vi "extract_XML_string_between_start_end-2.vi"(10 "type":string, 11 "XML_Cluster_String in":string) -> (0 "InTagDefines":T1(array[cluster]), 1 "XML_between_startANDEnd":string, 2 "nesting_level":i32, 3 "XML_after_start_end_pair":string)   [LabVIEW 2011]
doc: "This VI will return the content between a start and end demarkation in XML finding the appropriate pair even when nested within another of the same type. As and example\n\nhello not this\n<device>\n this\n <device>\n more more more\n </device>\n and this\n</device>\nnot this \n\nwill return:\n this\n <device>\n more more more\n </device>\n and this\n\n\nit will omit the start and end strings."
uses:
  <vilib>/regexp/Match Regular Expression.xnode
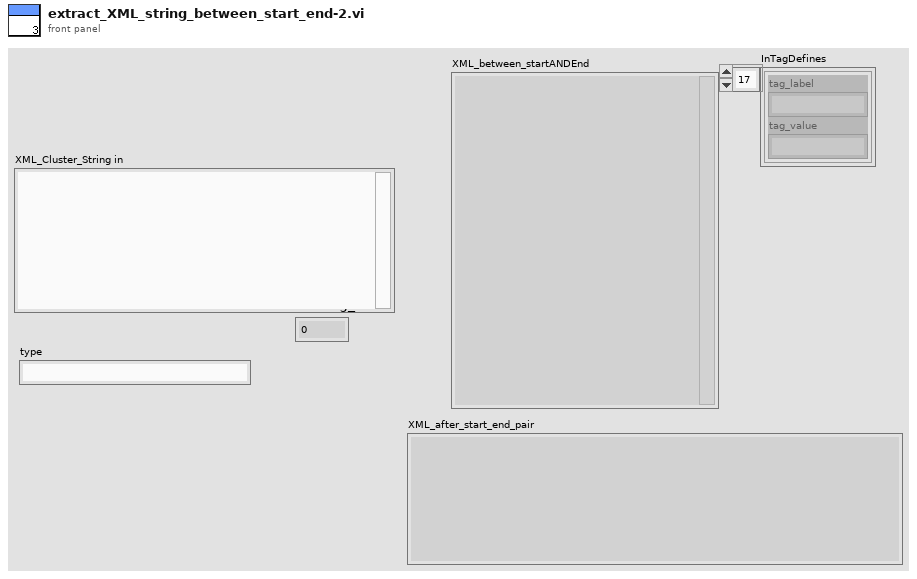
[diagram p1: front panel]
types:
  T1 = cluster{"tag_label":string, "tag_value":string}[]
  T2 = cluster{"submatch 1":string, "submatch 2":string}[]
  T3 = cluster{"submatch 1":string, "submatch 2":string}
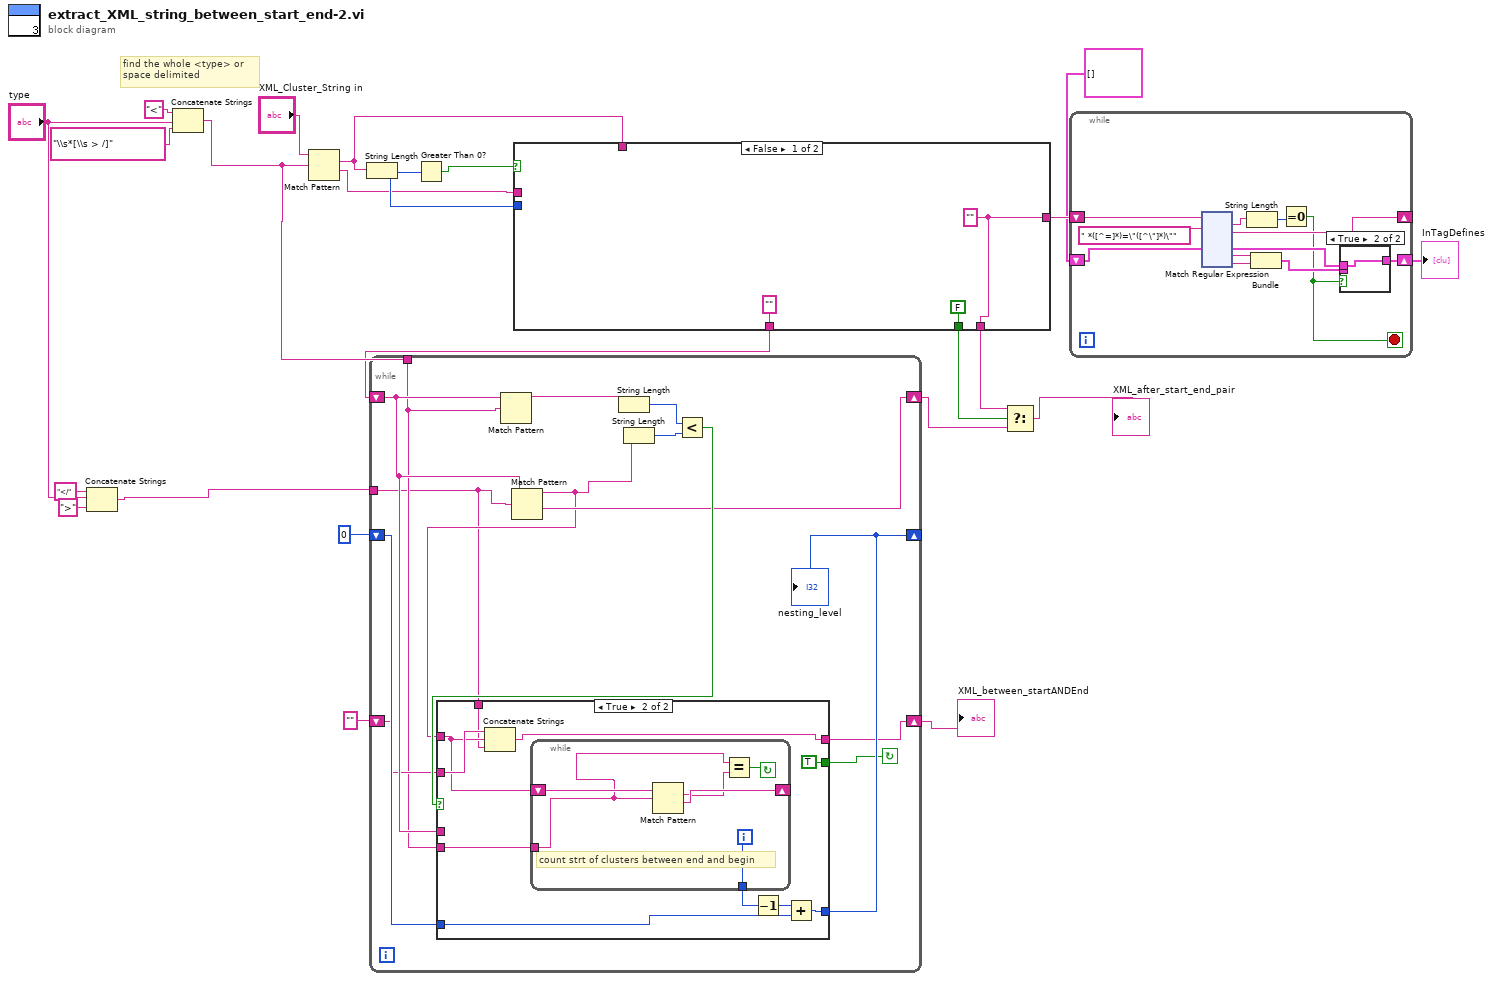
[diagram p0: block diagram]
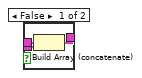
[diagram p2: hidden frame]
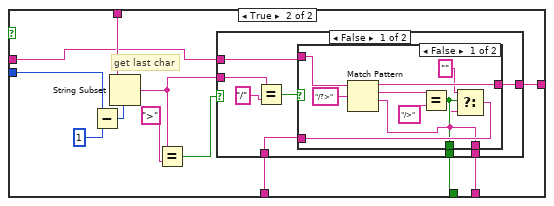
[diagram p3: hidden frame]
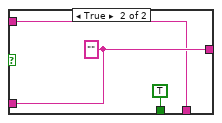
[diagram p4: hidden frame]
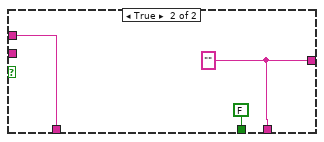
[diagram p5: hidden frame]
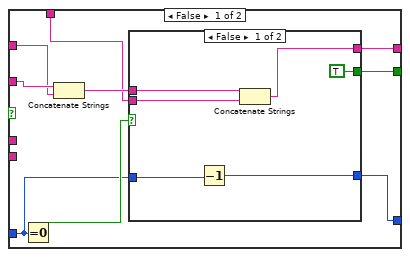
[diagram p6: hidden frame]
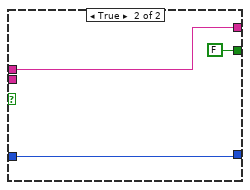
[diagram p7: hidden frame]
diagram:
  # "find the whole <type> or \nspace delimited"
  n1 = Concatenate Strings("</" ("string"), "type", ">" ("string")) -> (w21:string)
  n2 = Concatenate Strings("<" ("string"), "type", "\\s*[\\s > /]" ("string")) -> (w20:string)
  n3 = Match Pattern(string="XML_Cluster_String in", regular expression=w20) -> (match substring=w14:string, after substring=w9:string)  [unwired: 1 in, 2 out]
  n4 = String Length(string=w14) -> (length=w13:i32)
  n5 = Greater Than 0?(x=w13) -> (x > 0?=w10:bool)
  n6 = case shown="False" w10 {
    tunnel: w14 -> [_ w38]
    tunnel: w13 -> [_ w37]
    tunnel: w9 -> [_ w32]
    tunnel: ["" ("XML_Cluster_String in") w31] -> w8
    tunnel: [w24 w29] -> w7
    tunnel: [FALSE w28] -> w2
    tunnel: [w24 w27] -> w1
    frame False {
      w24 = "" ("XML_Cluster_String in")
    }
    frame True {
      # "get last char"
      n7 = Subtract(x=w37, y=1) -> (x-y=w35:i32)
      n8 = String Subset(string=w38, offset (0)=w35) -> (substring=w30:string)  [unwired: 1 in]
      n9 = Equal?(x=w30, y=">") -> (x = y?=w33:bool)
      n10 = case shown="False" w33 {
        tunnel: w32 -> [w44 w61]
        tunnel: [w43 w61] -> w31
        tunnel: w30 -> [w46 _]
        tunnel: [w42 w59] -> w29
        tunnel: [w40 FALSE] -> w28
        tunnel: [w39 w59] -> w27
        frame False {
          n11 = Equal?(x=w46, y="/") -> (x = y?=w41:bool)
          n12 = case shown="False" w41 {
            tunnel: w44 -> [w55 w56]
            tunnel: [w50 w58] -> w43
            tunnel: [w53 w58] -> w42
            tunnel: [w49 TRUE] -> w40
            tunnel: [w47 w56] -> w39
            frame False {
              n13 = Match Pattern(string=w55, regular expression="/?>") -> (before substring=w53:string, match substring=w52:string, after substring=w47:string)  [unwired: 1 in, 1 out]
              n14 = Equal?(x=w52, y="/>") -> (x = y?=w49:bool)
              n15 = Select(t="", s=w49, f=w47) -> (s? t:f=w50:string)
            }
            frame True {
              w58 = "" ("XML_Cluster_String in")
            }
          }
        }
        frame True {
          w59 = "" ("XML_Cluster_String in")
        }
      }
    }
  }
  n16 = while {
    shift-right: [w68] -> w3
    shift-left: w8 -> [w67]
    shift-right: [w70] -> _
    shift-left: 0 -> [w71]
    shift-right: [w64] -> w22
    shift-left: "" ("after substring") -> [w65]
    tunnel: w20 -> [w63]
    tunnel: w21 -> [w62]
    stop <- w69 continue-if-true
    n17 = Match Pattern(string=w67, regular expression=w63) -> (before substring=w75:string)  [unwired: 1 in, 3 out]
    n18 = Match Pattern(string=w67, regular expression=w62) -> (before substring=w66:string, after substring=w68:string)  [unwired: 1 in, 2 out]
    n19 = String Length(string=w75) -> (length=w74:i32)
    n20 = String Length(string=w66) -> (length=w73:i32)
    n21 = Less?(x=w74, y=w73) -> (x < y?=w72:bool)
    n22 = case shown="True" w72 {
      tunnel: w66 -> [w81 w99]
      tunnel: w71 -> [w78 w103]
      tunnel: [w77 w102] -> w70
      tunnel: [w83 TRUE] -> w69
      tunnel: w67 -> [_ _]
      tunnel: w65 -> [w82 w100]
      tunnel: [w79 w98] -> w64
      tunnel: w63 -> [_ w95]
      tunnel: w62 -> [w76 w94]
      frame False {
        n23 = Equal To 0?(x=w78) -> (x = 0?=w84:bool)
        n24 = Concatenate Strings(w82, w81) -> (w80:string)
        n25 = case shown="False" w84 {
          tunnel: [TRUE FALSE] -> w83
          tunnel: w80 -> [w90 w92]
          tunnel: [w89 w92] -> w79
          tunnel: w78 -> [w88 w91]
          tunnel: [w87 w91] -> w77
          tunnel: w76 -> [w85 _]
          frame False {
            n26 = Decrement(x=w88) -> (x-1=w87:i32)
            n27 = Concatenate Strings(w90, w85) -> (w89:string)
          }
          frame True {
          }
        }
      }
      frame True {
        n28 = Concatenate Strings(w100, w99, w94) -> (w98:string)
        n29 = while {
          shift-right: [w108] -> _
          shift-left: w99 -> [w109]
          tunnel: [w105] -> w97
          tunnel: w95 -> [w104]
          i -> [w105]
          stop <- w106 continue-if-true
          # "count strt of clusters between end and begin"
          n30 = Match Pattern(string=w109, regular expression=w104) -> (match substring=w107:string, after substring=w108:string)  [unwired: 1 in, 2 out]
          n31 = Equal?(x=w104, y=w107) -> (x = y?=w106:bool)
        }
        n32 = Decrement(x=w97) -> (x-1=w96:i32)
        n33 = Add(x=w96, y=w103) -> (x+y=w102:i32)
      }
    }
    "nesting_level" <- w70
  }
  "XML_between_startANDEnd" <- w22
  n34 = Select(t=w1, s=w2, f=w3) -> (s? t:f=→"XML_after_start_end_pair":string)
  n35 = while {
    shift-right: [w116] -> _
    shift-left: w7 -> [w120]
    shift-right: [w113] -> w6
    shift-left: T2 [] -> [w111]
    stop <- w110 stop-if-true
    n36 = xnode "Match Regular Expression"("input string"=w120, "regular expression"=" *([^=]*)=\"([^\"]*)\"") -> ("whole match"=w115:string, "after match"=w116:string, "submatch 1"=w118:string, "submatch 2"=w117:string)  [unwired: 4 in, 3 out]
    n37 = String Length(string=w115) -> (length=w114:i32)
    n38 = Bundle("submatch 1"=w118, "submatch 2"=w117) -> (w112:T3)  [unwired: 1 in]
    n39 = Equal To 0?(x=w114) -> (x = 0?=w110:bool)
    n40 = case shown="True" w110 {
      tunnel: [w123 w124] -> w113
      tunnel: w112 -> [w122 _]
      tunnel: w111 -> [w121 w124]
      frame False {
        n41 = Build Array (concatenate)(w121, w122) -> (w123:T2)
      }
      frame True {
      }
    }
  }
  "InTagDefines" <- w6
